vi "IND560 Select Station.vi"(11 "All Stations":T1[](array[typedef])) -> (2 "IND560 Selector 2":T1)   [LabVIEW 2020]
uses:
  Type Definitions/IND560 Data Output Selector.ctl
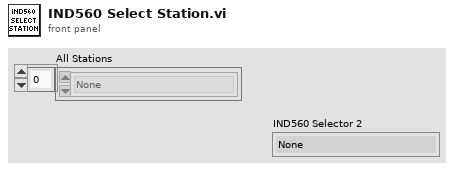
[diagram p1: front panel]
types:
  T1 = typedef "IND560 Data Output Selector.ctl" = enum16{"None", "Use Gross Not Equal Net", "Use Gross Equal Net", "Use Unstable Weights"}
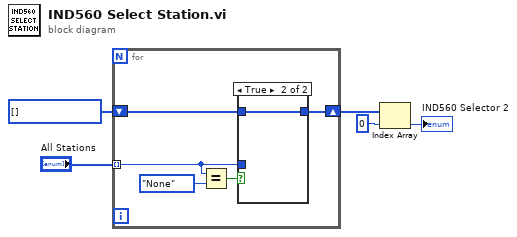
[diagram p0: block diagram]
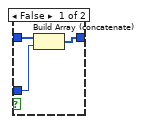
[diagram p2: hidden frame]
diagram:
  w2 = T1[] [] items=["None", "Use Gross Not Equal Net", "Use Gross Equal Net", "Use Unstable Weights"]
  n1 = for {
    tunnel: "All Stations" -> [w6] mode=indexing
    shift-right: [w7] -> w3
    shift-left: w2 -> [w8]
    n2 = Equal?(x=w6, y=IND560_Data_Output_Selector."None") -> (x = y?=w10:bool)
    n3 = case shown="True" w10 {
      tunnel: w8 -> [w13 w14]
      tunnel: [w12 w14] -> w7
      tunnel: w6 -> [w11 _]
      frame False {
        n4 = Build Array (concatenate)(w13, w11) -> (w12:T1[])
      }
      frame True {
      }
    }
  }
  n5 = Index Array(array=w3, index=0) -> (element=→"IND560 Selector 2":T1)
